vi "Send Std to DAQ.vi"(6 "Just send!":bool, 8 "error in (no error)":errorcluster, 9 "New Message":string, 10 "Std Selector":T1, 11 "Kasli Wrapper 2.0 in":refnum<class "Kasli Wrapper 2.0.lvclass">=refnum) -> (0 "error out":errorcluster, 3 "Kasli Wrapper 2.0 out":refnum<class "Kasli Wrapper 2.0.lvclass">)   [LabVIEW 2020, in "CIRCUS_uServices.lvlib" / "Kasli Wrapper 2.0.lvlib" / "Kasli Wrapper 2.0.lvclass"]
doc: "This VI sends the Std logs to the DAQ, but in bunches of N messages (10). \nIt maintains a buffer of messages to which New Message is appended, and if the buffer is long enough, it clears it and send it to the DAQ.\nIf Just send! is True, then the buffer is sent to the DAQ independently from its size."
uses:
  Kasli Wrapper 2.0.lvclass
  TALOS/TALOS_PPL.lvlibp/Father of all uServices/Father of all uServices/Father of all uServices.lvclass
  TALOS/TALOS_PPL.lvlibp
  C:/Users/marco/Documents/GitHub_Lab/CIRCUS/TALOS/TALOS_PPL.lvlibp/Ancestor/Ancestor/Ancestor.lvclass
  C:/Users/marco/Documents/GitHub_Lab/CIRCUS/TALOS/Actor Framework.lvlibp/1abvi3w/vi.lib/ActorFramework/Actor/Actor.lvclass
  C:/Users/marco/Documents/GitHub_Lab/CIRCUS/TALOS/TALOS_PPL.lvlibp/Father of all uServices/Father of all uServices/Father of all uServices.lvclass
  Std Selector.ctl
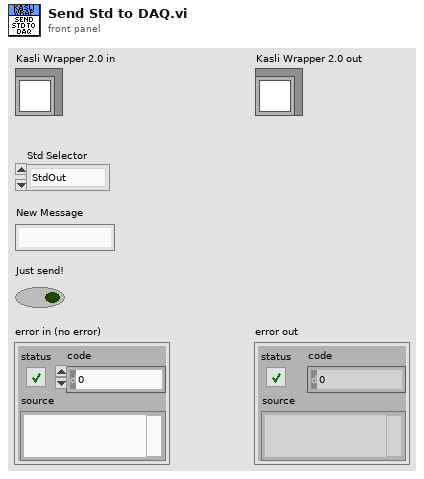
[diagram p1: front panel]
types:
  T1 = typedef "CIRCUS_uServices.lvlib/Kasli Wrapper 2.0.lvlib/Kasli Wrapper 2.0.lvclass/Std Selector.ctl" = enum16{"StdOut", "StdErr"}
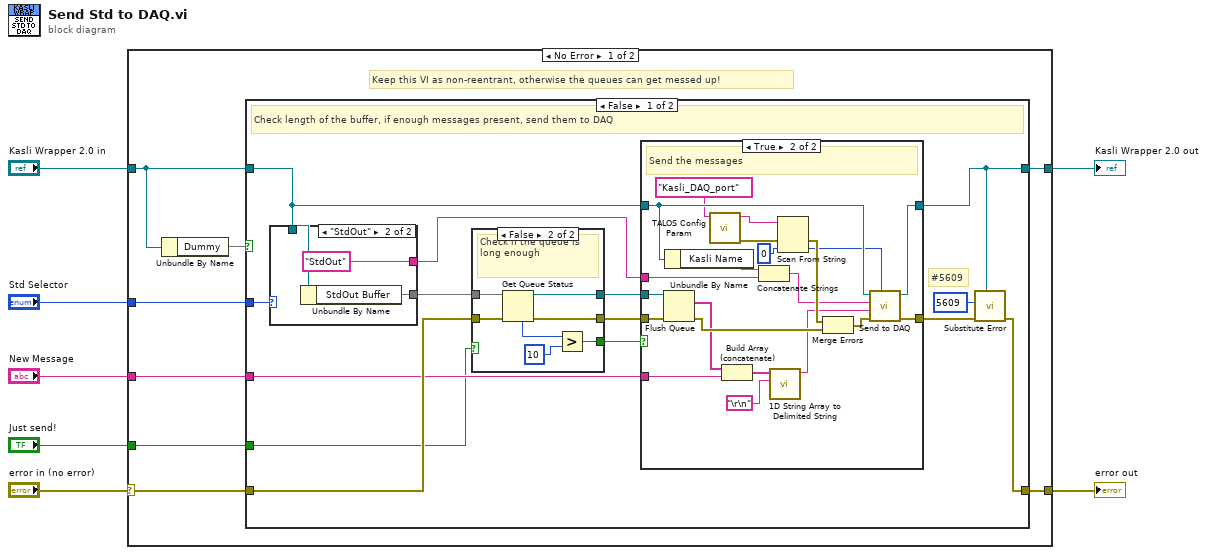
[diagram p0: block diagram]
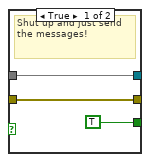
[diagram p2: hidden frame]
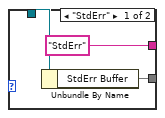
[diagram p3: hidden frame]
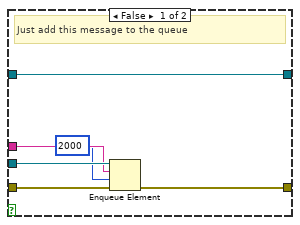
[diagram p4: hidden frame]
diagram:
  n1 = case shown="No Error" "error in (no error)" {
    selector: "error in (no error)" -> [w14 w75]
    tunnel: "Kasli Wrapper 2.0 in" -> [w13 w76]
    tunnel: "Std Selector" -> [w15 _]
    tunnel: [w11 w76] -> w4
    tunnel: [w10 w75] -> w3
    tunnel: "New Message" -> [w9 _]
    tunnel: "Just send!" -> [w8 _]
    frame No Error {
      # "Keep this VI as non-reentrant, otherwise the queues can get messed up!"
      n2 = Unbundle By Name(w13) -> ("Dummy"=w12)
      n3 = case shown="False" w12 {
        tunnel: w15 -> [w29 _]
        tunnel: w14 -> [w28 w73]
        tunnel: w13 -> [w26 w74]
        tunnel: [w17 w74] -> w11
        tunnel: [w18 w73] -> w10
        tunnel: w9 -> [w27 _]
        tunnel: w8 -> [w21 _]
        frame False {
          # "#5609"
          # "Check length of the buffer, if enough messages present, send them to DAQ"
          n4 = case shown="\"StdOut\"" w29 {
            tunnel: [w42 w45] -> w24
            tunnel: w26 -> [w41 w44]
            tunnel: ["StdErr" "StdOut"] -> w25
            frame "StdErr" {
              n5 = Unbundle By Name(w41) -> ("StdErr Buffer"=w42)
            }
            frame "StdOut" {
              n6 = Unbundle By Name(w44) -> ("StdOut Buffer"=w45)
            }
          }
          n7 = case shown="False" w21 {
            tunnel: w28 -> [w31 w39]
            tunnel: w24 -> [w32 w36]
            tunnel: [w32 w35] -> w23
            tunnel: [w31 w34] -> w22
            tunnel: [TRUE w33] -> w20
            frame True {
              # "Shut up and just send the messages!"
            }
            frame False {
              # "Check if the queue is long enough"
              n8 = Get Queue Status(queue=w36, error in (no error)=w39) -> (queue out=w35:refnum<queue>, error out=w34:errorcluster, # elements in queue=w38:i32)  [unwired: 1 in, 5 out]
              n9 = Greater?(x=w38, y=10) -> (0:w33:bool)
            }
          }
          n10 = case shown="True" w20 {
            tunnel: w23 -> [w50 w70]
            tunnel: w27 -> [_ w68]
            tunnel: w26 -> [w51 w60]
            tunnel: w25 -> [w49 w66]
            tunnel: w22 -> [w47 w65]
            tunnel: [w51 w59] -> w17
            tunnel: [w46 w58] -> w19
            frame False {
              # "Just add this message to the queue"
              n11 = Enqueue Element(queue=w50, element=w49, timeout in ms (-1)=2000, error in (no error)=w47) -> (error out=w46:errorcluster)  [unwired: 2 out]
            }
            frame True {
              # "Send the messages"
              n12 = Flush Queue(queue=w70, error in (no error)=w65) -> (remaining elements=w69:string[], error out=w71:errorcluster)  [unwired: 1 out]
              n13 = Unbundle By Name(w60) -> ("Kasli Name"=w67)
              n14 = call "TALOS Config Param.vi"("Parameter Name"="Kasli_DAQ_port") -> ("error out"=w56:errorcluster, "Output"=w55:string)  [unwired: 9 in]
              n15 = Build Array (concatenate)(w69, w68) -> (w64:string[])
              n16 = Concatenate Strings(w67, w66) -> (w61:string)
              n17 = call <vilib>:"1D String Array to Delimited String.vi"("delimiter"="\r\n", "string array"=w64) -> ("delimited string"=w62:string)  [unwired: 9 in]
              n18 = Scan From String(input string=w55, error in=w56, default 1=u16 0) -> (error out=w72:errorcluster, output 1=w53:u16)  [unwired: 2 in, 2 out]
              n19 = Merge Errors(w72, w71) -> (w52:errorcluster)
              n20 = call "Send to DAQ.vi"("Port Number"=w53, "error in (no error)"=w52, "Data"=w62, "Data Name"=w61, "Father of all uServices in"=w60) -> ("error out"=w58:errorcluster, "Father of all uServices out"=w59:refnum<class "Father of all uServices.lvclass">)  [unwired: 5 in]
            }
          }
          n21 = call "Substitute Error.vi"("LabVIEW Object"=w17, "error in (no error)"=w19, "Error Code"=5609) -> ("error out"=w18:errorcluster)  [unwired: 8 in]
        }
        frame True {
          # "If Dummy we don't send anything to the DAQ!"
        }
      }
    }
    frame Error {
    }
  }
  "error out" <- w3
  "Kasli Wrapper 2.0 out" <- w4
